vi "SV TDMS Read Unit Info.vi"(0 "tdms file":refnum<k34>, 5 "group name":string, 7 "channel name":string, 11 "error in (no error)":errorcluster) -> (4 "tdms file out":refnum<k34>, 6 "group name out":string, 8 "channel name out":string, 13 "scale labels":T1, 14 "unit info":T2, 15 "error out":errorcluster)   [LabVIEW 2017]
uses:
  <vilib>/addons/_NISVFA/_Shared subVIs/Controls/svc_Unit Info.ctl
  <vilib>/addons/_NISVFA/_Shared subVIs/Controls/NI Channel Properties.ctl
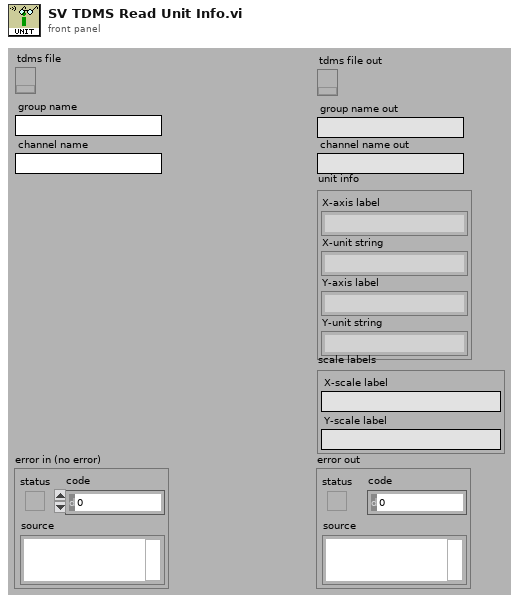
[diagram p1: front panel]
types:
  T1 = cluster{"X-scale label":string, "Y-scale label":string}
  T2 = typedef "svc_Unit Info.ctl" = cluster{"X-axis label":string, "X-unit string":string, "Y-axis label":string, "Y-unit string":string}
  T3 = typedef "NI Channel Properties.ctl" = u16
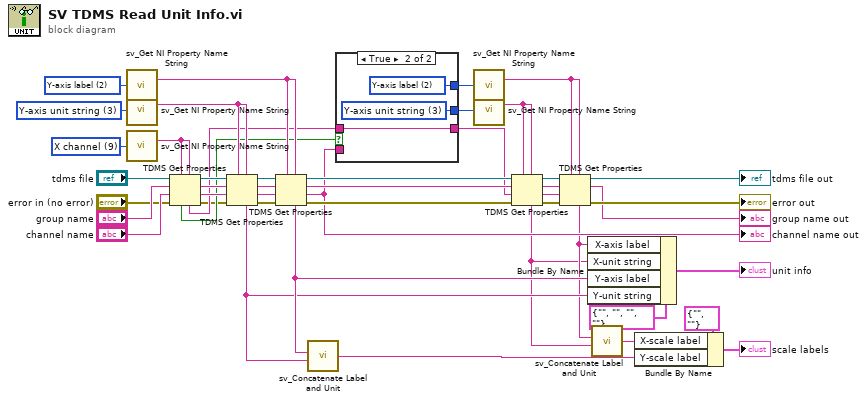
[diagram p0: block diagram]
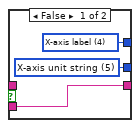
[diagram p2: hidden frame]
diagram:
  w23 = T3 9 items=["Channel name", "Channel description", "Y-axis label", "Y-axis unit string", "X-axis label", "X-axis unit string", "x0", "dx", "Number of samples", "X channel", "Filter settled", "dB reference", "Window", "Window parameter", "Window size", "FFT size", "Peak units", "Spectrum type", "Magnitude scale", "Spectral density", "Sensor sensitivity (mV/EU)", "X-axis domain", "LabVIEW datatype"] ("property")
  w41 = T3 3 items=["Channel name", "Channel description", "Y-axis label", "Y-axis unit string", "X-axis label", "X-axis unit string", "x0", "dx", "Number of samples", "X channel", "Filter settled", "dB reference", "Window", "Window parameter", "Window size", "FFT size", "Peak units", "Spectrum type", "Magnitude scale", "Spectral density", "Sensor sensitivity (mV/EU)", "X-axis domain", "LabVIEW datatype"] ("property")
  w42 = T3 2 items=["Channel name", "Channel description", "Y-axis label", "Y-axis unit string", "X-axis label", "X-axis unit string", "x0", "dx", "Number of samples", "X channel", "Filter settled", "dB reference", "Window", "Window parameter", "Window size", "FFT size", "Peak units", "Spectrum type", "Magnitude scale", "Spectral density", "Sensor sensitivity (mV/EU)", "X-axis domain", "LabVIEW datatype"] ("property")
  n1 = call <vilib>:"sv_Get NI Property Name String.vi"("property"=w42) -> ("TDMS property name"=w28:string)  [unwired: 13 in, 1 out]
  n2 = call <vilib>:"sv_Get NI Property Name String.vi"("property"=w41) -> ("TDMS property name"=w29:string)  [unwired: 13 in, 1 out]
  n3 = call <vilib>:"sv_Get NI Property Name String.vi"("property"=w23) -> ("TDMS property name"=w20:string)  [unwired: 13 in, 1 out]
  n4 = TDMS Get Properties(5:w20, 7:w20, 8:"error in (no error)", 9:"channel name", 10:"group name", 11:"tdms file") -> (0:w6:errorcluster, 1:w14:string, 2:w21:string, 3:w18:refnum<k34>, 4:w11:string, 6:w13:bool)
  n5 = TDMS Get Properties(5:w29, 7:w29, 8:w6, 9:w14, 10:w21, 11:w18) -> (0:w46:errorcluster, 1:w45:string, 2:w44:string, 3:w43:refnum<k34>, 4:w16:string)  [unwired: 1 out]
  n6 = TDMS Get Properties(5:w28, 7:w28, 8:w46, 9:w45, 10:w44, 11:w43) -> (0:w36:errorcluster, 1:w9:string, 2:w35:string, 3:w12:refnum<k34>, 4:w17:string)  [unwired: 1 out]
  "channel name out" <- w9
  n7 = call <vilib>:"sv_Concatenate Label and Unit.vi"("unit string"=w16, "label"=w17) -> ("scale label with units"=w15:string)  [unwired: 4 in]
  n8 = case shown="True" w13 {
    tunnel: [w49 w52] -> w31
    tunnel: [w48 w51] -> w30
    tunnel: w9 -> [w47 _]
    tunnel: w11 -> [_ w50]
    tunnel: [w47 w50] -> w10
    frame False {
      w48 = T3 5 items=["Channel name", "Channel description", "Y-axis label", "Y-axis unit string", "X-axis label", "X-axis unit string", "x0", "dx", "Number of samples", "X channel", "Filter settled", "dB reference", "Window", "Window parameter", "Window size", "FFT size", "Peak units", "Spectrum type", "Magnitude scale", "Spectral density", "Sensor sensitivity (mV/EU)", "X-axis dimension", "LabVIEW datatype", "Function type", "Function subtype", "X values", "Independent channel"] ("property")
      w49 = T3 4 items=["Channel name", "Channel description", "Y-axis label", "Y-axis unit string", "X-axis label", "X-axis unit string", "x0", "dx", "Number of samples", "X channel", "Filter settled", "dB reference", "Window", "Window parameter", "Window size", "FFT size", "Peak units", "Spectrum type", "Magnitude scale", "Spectral density", "Sensor sensitivity (mV/EU)", "X-axis dimension", "LabVIEW datatype", "Function type", "Function subtype", "X values", "Independent channel"] ("property")
    }
    frame True {
      w51 = T3 3 items=["Channel name", "Channel description", "Y-axis label", "Y-axis unit string", "X-axis label", "X-axis unit string", "x0", "dx", "Number of samples", "X channel", "Filter settled", "dB reference", "Window", "Window parameter", "Window size", "FFT size", "Peak units", "Spectrum type", "Magnitude scale", "Spectral density", "Sensor sensitivity (mV/EU)", "X-axis domain", "LabVIEW datatype"] ("property")
      w52 = T3 2 items=["Channel name", "Channel description", "Y-axis label", "Y-axis unit string", "X-axis label", "X-axis unit string", "x0", "dx", "Number of samples", "X channel", "Filter settled", "dB reference", "Window", "Window parameter", "Window size", "FFT size", "Peak units", "Spectrum type", "Magnitude scale", "Spectral density", "Sensor sensitivity (mV/EU)", "X-axis domain", "LabVIEW datatype"] ("property")
    }
  }
  n9 = call <vilib>:"sv_Get NI Property Name String.vi"("property"=w31) -> ("TDMS property name"=w26:string)  [unwired: 13 in, 1 out]
  n10 = call <vilib>:"sv_Get NI Property Name String.vi"("property"=w30) -> ("TDMS property name"=w27:string)  [unwired: 13 in, 1 out]
  n11 = TDMS Get Properties(5:w27, 7:w27, 8:w36, 9:w10, 10:w35, 11:w12) -> (0:w37:errorcluster, 1:w38:string, 2:w39:string, 3:w40:refnum<k34>, 4:w4:string)  [unwired: 1 out]
  n12 = TDMS Get Properties(5:w26, 7:w26, 8:w37, 9:w38, 10:w39, 11:w40) -> (0:→"error out":errorcluster, 2:→"group name out":string, 3:→"tdms file out":refnum<k34>, 4:w5:string)  [unwired: 2 out]
  n13 = Bundle By Name(cluster=T2 {"X-axis label"="", "X-unit string"="", "Y-axis label"="", "Y-unit string"=""} ("unit info 2"), "X-axis label"=w5, "X-unit string"=w4, "Y-axis label"=w17, "Y-unit string"=w16) -> (→"unit info":T2)
  n14 = call <vilib>:"sv_Concatenate Label and Unit.vi"("unit string"=w4, "label"=w5) -> ("scale label with units"=w3:string)  [unwired: 4 in]
  n15 = Bundle By Name(cluster=T1 {"X-scale label"="", "Y-scale label"=""} ("scale labels"), "X-scale label"=w3, "Y-scale label"=w15) -> (→"scale labels":T1)
